vi "genGroove.vi"(9 "Depth":dbl=-1.0, 10 "Groove Length":dbl=3.0, 11 "armID":i32) -> (0 "zVisTraj":dbl[](array[numeric]) format="%_6g", 1 "yVisTraj":dbl[](array[numeric]) format="%_6g", 2 "xVisTraj":dbl[](array[numeric]) format="%_6g")   [LabVIEW 2016]
uses:
  <vilib>/Math Plots/3D Math Plots/3D Scatter/3D Scatter Datatype/3D Scatter Datatype.lvclass
  <vilib>/gmath/NI_Gmath.lvlib
  <vilib>/Analysis/NI_AALBase.lvlib
  <vilib>/Analysis/1siggen.llb/Ramp Pattern by Samples.vi
  <vilib>/Math Plots/3D Math Plots/3D Scatter/3D Scatter Datatype/Public/Plot Helper (Vector).vi
  <vilib>/Math Plots/3D Math Plots/3D Scatter/3D Scatter XCtrl/3D Scatter.xctl
panel:
  out "Trajectory OOB":bool
  in  "joint limits":dbl[][](array[numeric])=[[-68.0, -4.0], [-35.0, 35.0], [0.1, 10.0], [-40.0, 40.0]]
  out "size(s)":i32
  out "Groove Plot":refnum<class "3D Plot Datatype.lvclass">[](xcontrol)
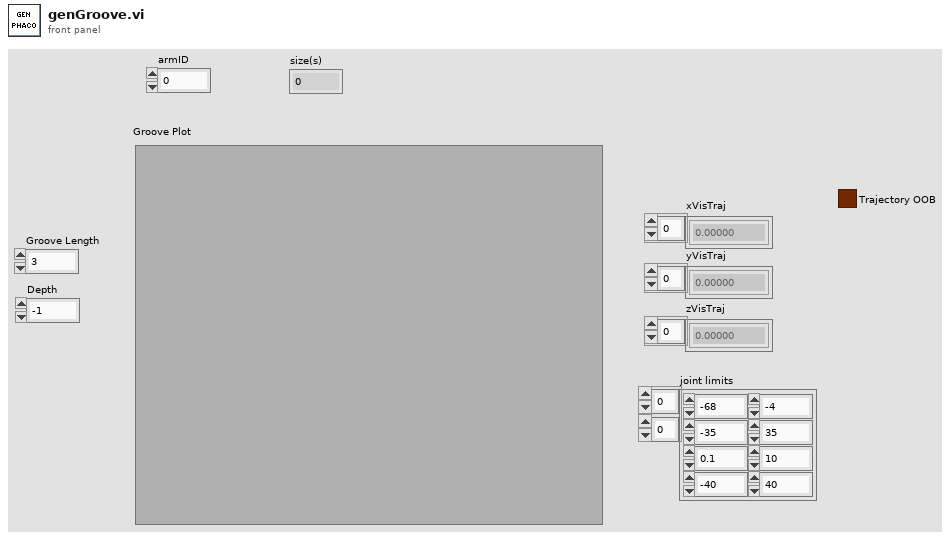
[diagram p1: front panel]
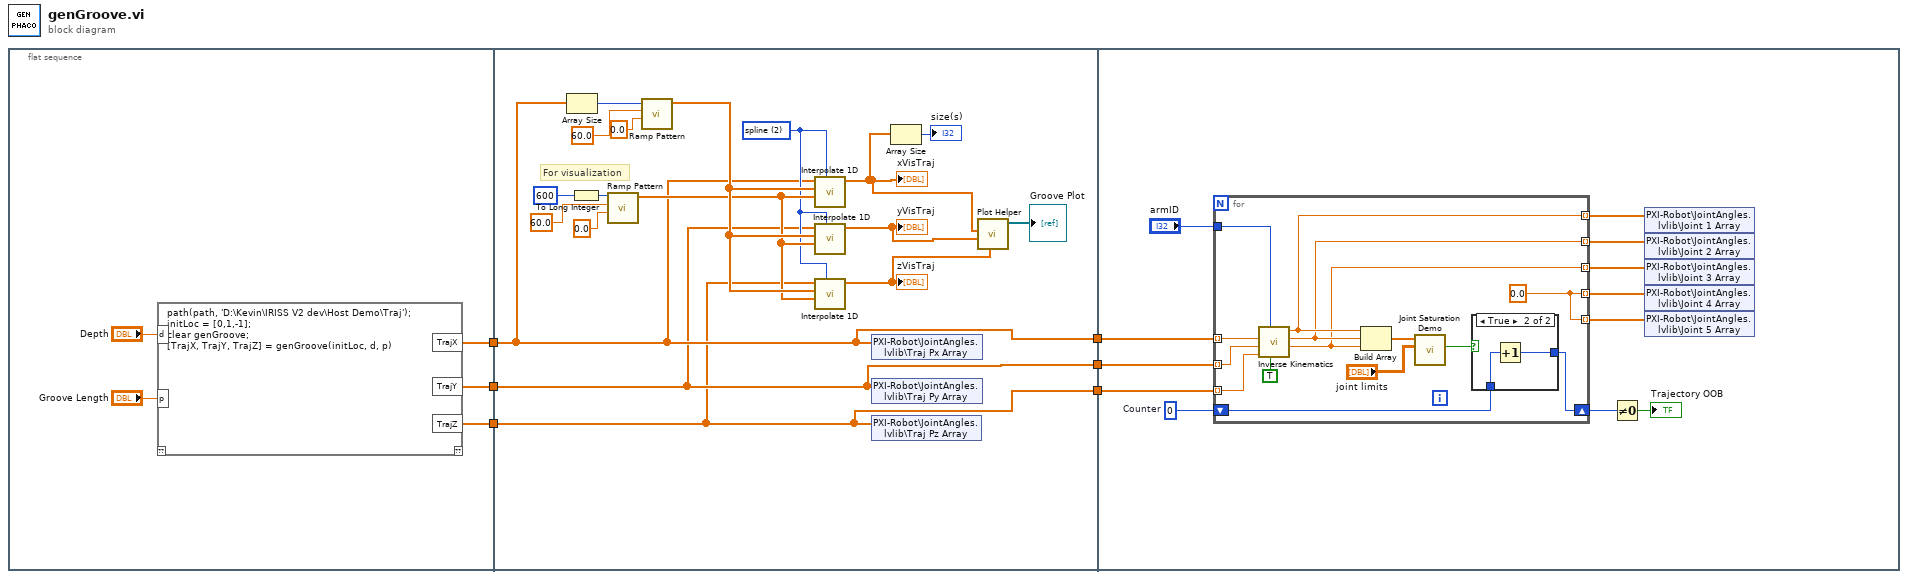
[diagram p0: block diagram]
diagram:
  n1 = flat-sequence {
    tunnel: [w9] -> w6
    tunnel: [w8] -> w5
    tunnel: [w7] -> w4
    tunnel: w6 -> [w16]
    tunnel: w5 -> [w15]
    tunnel: w4 -> [w17]
    tunnel: [w17] -> w3
    tunnel: [w16] -> w2
    tunnel: [w15] -> w1
    tunnel: w3 -> [w40]
    tunnel: w2 -> [w39]
    tunnel: w1 -> [w38]
    frame #0 {
      n2 = script code="path(path, 'D:\\Kevin\\IRISS V2 dev\\Host Demo\\Traj'); \ninitLoc = [0,1,-1]; \nclear genGroove;\n[TrajX, TrajY, TrajZ] = genGroove(initLoc, d, p)"("d"="Depth", "p"="Groove Length") -> ("TrajX"=w7:dbl[], "TrajY"=w9:dbl[], "TrajZ"=w8:dbl[])  [unwired: 1 in, 1 out]
    }
    frame #1 {
      w19 = 2 items=["nearest", "linear", "spline", "cubic Hermite", "Lagrange"] ("method")
      # "For visualization"
      n3 = Array Size(array=w17) -> (size(s)=w26:i32)
      n4 = To Long Integer(number=600) -> (32bit integer=w20:i32)
      n5 = call-poly <vilib>:"Ramp Pattern.vi"("start"=0.0, "end"=60.0, "samples"=w20) -> ("Ramp Pattern"=w22:dbl[])  [unwired: 7 in, 1 out]
      n6 = call-poly <vilib>:"Ramp Pattern.vi"("start"=0.0, "end"=60.0, "samples"=w26) -> ("Ramp Pattern"=w27:dbl[])  [unwired: 7 in, 1 out]
      n7 = call <vilib>:"Interpolate 1D.vi"("method"=w19, "xi"=w22, "X"=w27, "Y"=w17) -> ("yi"=w14:dbl[])  [unwired: 5 in, 2 out]
      "xVisTraj" <- w14
      n8 = call <vilib>:"Interpolate 1D.vi"("method"=w19, "xi"=w22, "X"=w27, "Y"=w16) -> ("yi"=w13:dbl[])  [unwired: 5 in, 2 out]
      "yVisTraj" <- w13
      n9 = call <vilib>:"Interpolate 1D.vi"("method"=w19, "xi"=w22, "X"=w27, "Y"=w15) -> ("yi"=w12:dbl[])  [unwired: 5 in, 2 out]
      "zVisTraj" <- w12
      n10 = shared-variable "PXI-Robot\\JointAngles.lvlib\\Traj Px Array"(w17) -> ()  [unwired: 1 in, 1 out]
      n11 = shared-variable "PXI-Robot\\JointAngles.lvlib\\Traj Py Array"(w16) -> ()  [unwired: 1 in, 1 out]
      n12 = shared-variable "PXI-Robot\\JointAngles.lvlib\\Traj Pz Array"(w15) -> ()  [unwired: 1 in, 1 out]
      n13 = Array Size(array=w14) -> (size(s)=→"size(s)":i32)
      n14 = call-poly <vilib>:"Plot Helper.vi"("z vector"=w12, "y vector"=w13, "x vector"=w14) -> ("3D Plot lvclass Array out"=→"Groove Plot":refnum<class "3D Plot Datatype.lvclass">[])  [unwired: 3 in, 5 out]
    }
    frame #2 {
      w37 = 0  # Counter
      n15 = for {
        tunnel: "armID" -> [w55]
        tunnel: w40 -> [w54] mode=indexing
        tunnel: w39 -> [w53] mode=indexing
        tunnel: w38 -> [w52] mode=indexing
        shift-right: [w47] -> w35
        shift-left: w37 -> [w48]
        tunnel: [w46] -> w34 mode=indexing
        tunnel: [w45] -> w33 mode=indexing
        tunnel: [w44] -> w32 mode=indexing
        tunnel: [w43] -> w30 mode=indexing
        tunnel: [w43] -> w31 mode=indexing
        w43 = 0.0 ("Numeric")
        n16 = call "Inverse Kinematics.vi"(6:TRUE ("isToolTipInsideEye"), "armID"=w55, "z"=w52, "y"=w53, "x"=w54) -> ("j3"=w44:dbl, "j2"=w45:dbl, "j1"=w46:dbl)  [unwired: 3 in, 1 out]
        n17 = Build Array(w46, w45, w44) -> (w50:dbl[])
        n18 = call "Joint Saturation Demo.vi"("Joint Bounds [Deg/mm]"="joint limits", "Ref Array [Deg/mm]"=w50) -> ("Out of Bound?"=w49:bool)  [unwired: 8 in, 1 out]
        n19 = case shown="True" w49 {
          tunnel: w48 -> [w56 w58]
          tunnel: [w56 w57] -> w47
          frame False {
          }
          frame True {
            n20 = Increment(x=w58) -> (x+1=w57:i32)
          }
        }
      }
      n21 = Not Equal To 0?(x=w35) -> (x != 0?=→"Trajectory OOB":bool)
      n22 = shared-variable "PXI-Robot\\JointAngles.lvlib\\Joint 1 Array"(w34) -> ()  [unwired: 1 in, 1 out]
      n23 = shared-variable "PXI-Robot\\JointAngles.lvlib\\Joint 2 Array"(w33) -> ()  [unwired: 1 in, 1 out]
      n24 = shared-variable "PXI-Robot\\JointAngles.lvlib\\Joint 3 Array"(w32) -> ()  [unwired: 1 in, 1 out]
      n25 = shared-variable "PXI-Robot\\JointAngles.lvlib\\Joint 4 Array"(w31) -> ()  [unwired: 1 in, 1 out]
      n26 = shared-variable "PXI-Robot\\JointAngles.lvlib\\Joint 5 Array"(w30) -> ()  [unwired: 1 in, 1 out]
    }
  }
